vi "Test Database API.vi"() -> ()   [LabVIEW 2016]
doc: "Database API Tester."
uses:
  Class/DB/Credential.ctl
  Class/DB/Update Credential.ctl
  <vilib>/Utility/error.llb/DialogType.ctl
  Database.lvlib
panel:
  in  "REQ Retry DB":bool
  in  "REQ Close DB Ref":bool
  in  "User Level":enum16{"Administrator", "Engineer", "Operator"}(ring)
  out "Username":string[](array[string])
  in  "REQ Get Username":bool
  out "Test Data Out":string[][](array[string])
  in  "To":timestamp
  in  "From":timestamp
  in  "REQ Load Test Data":bool
  in  "Test Data":string[](array[string])
  in  "REQ Save Test Data":bool
  in  "REQ Save DB Record Data":bool
  in  "REQ Delete Table Data":bool
  in  "List Table":string(combo)
  in  "REQ List Table":bool
  in  "New Credential":T1
  in  "REQ Update User Details":bool
  in  "REQ Delete User":bool
  out "Match?":bool
  in  "REQ Check Credential":bool
  in  "Credential":T2
  in  "REQ Add User":bool
  in  "Show Diagram on Init":bool
  in  "Show Block Diagram":bool
  in  "Stop Module":bool
  in  "Start Module":bool
  in  "Hide Module Panel":bool
  in  "Show Module Panel":bool
  out "Status":string
  out "Module Running?":bool
  # "This VI tests the API for the Module."
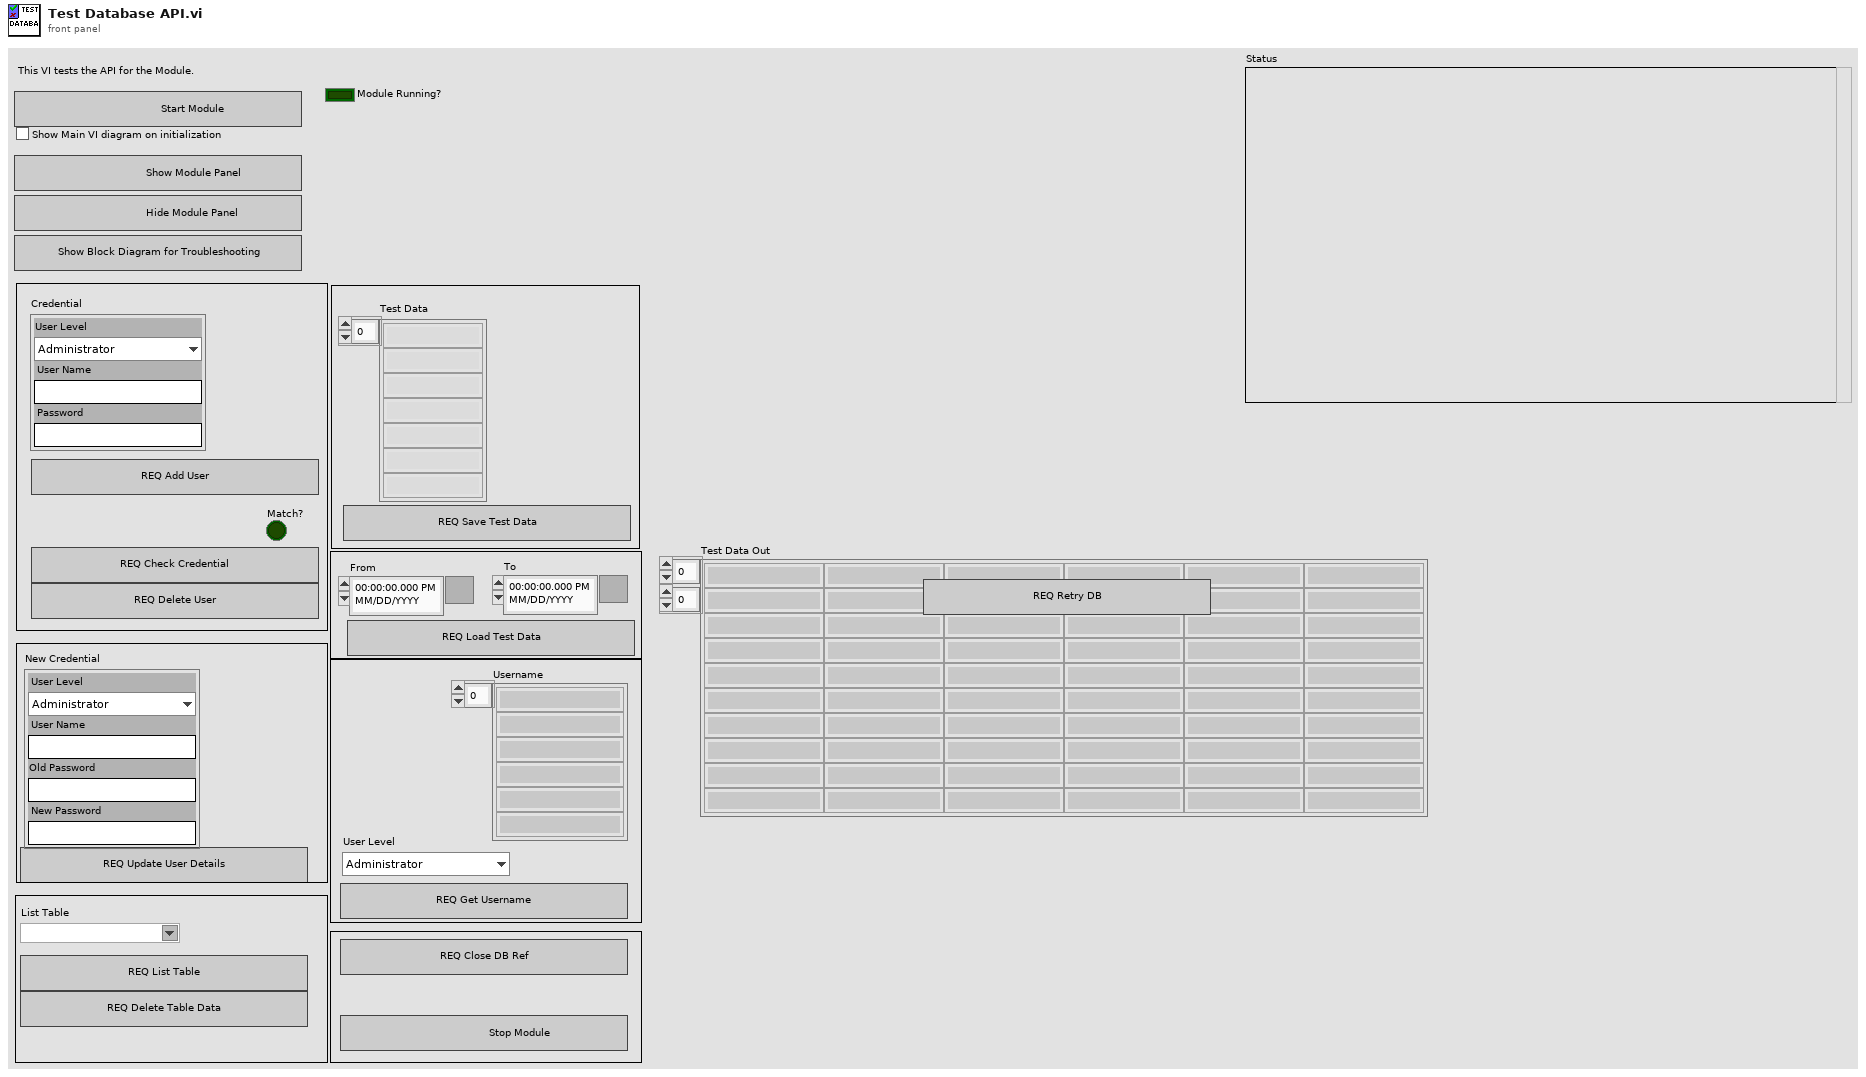
[diagram p1: front panel]
types:
  T1 = typedef "Database.lvlib/Update Credential.ctl" = cluster{"User Level":enum16{"Administrator", "Engineer", "Operator"}, "User Name":string, "Old Password":string, "New Password":string}
  T2 = typedef "Database.lvlib/Credential.ctl" = cluster{"User Level":enum16{"Administrator", "Engineer", "Operator"}, "User Name":string, "Password":string}
  T3 = typedef "Database.lvlib/Broadcast Events--cluster.ctl" = cluster{"Module Did Init":refnum<user-event>, "Status Updated":refnum<user-event>, "Error Reported":refnum<user-event>, "Module Did Stop":refnum<user-event>, "Update Module Execution Status":refnum<user-event>}
  T4 = typedef "DialogType.ctl" = u16
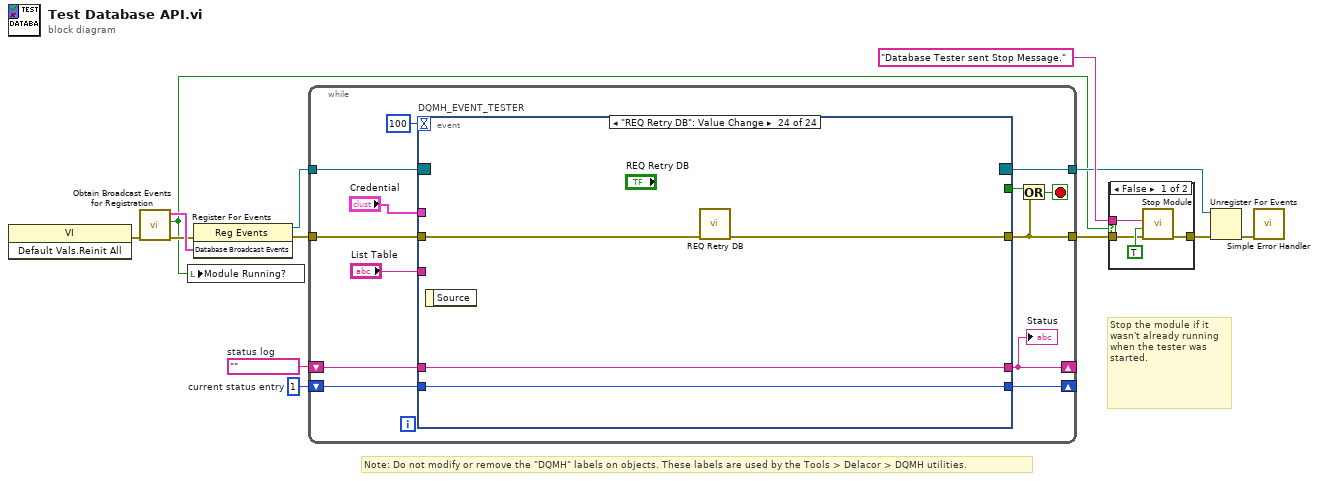
[diagram p0: block diagram]
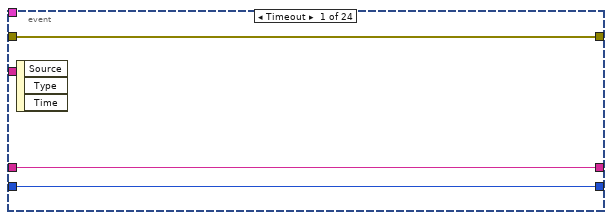
[diagram p3: hidden frame]
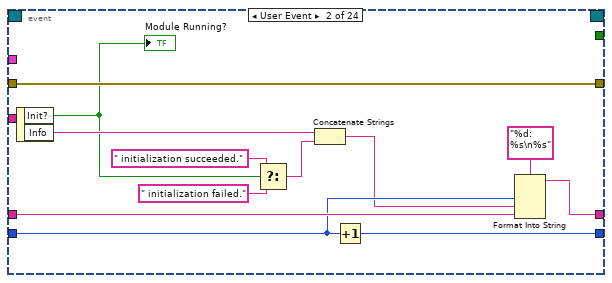
[diagram p4: hidden frame]
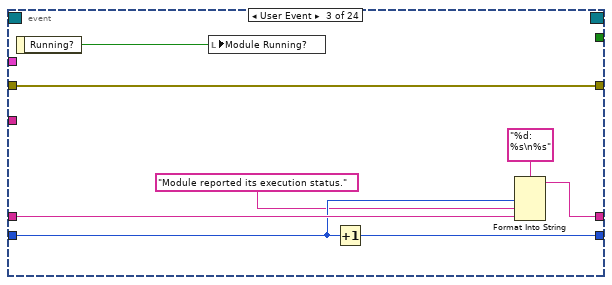
[diagram p5: hidden frame]
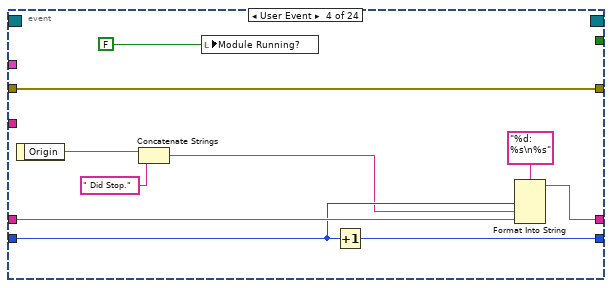
[diagram p6: hidden frame]
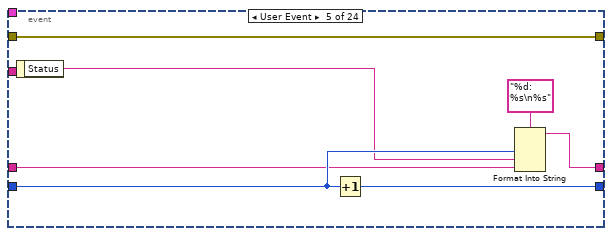
[diagram p7: hidden frame]
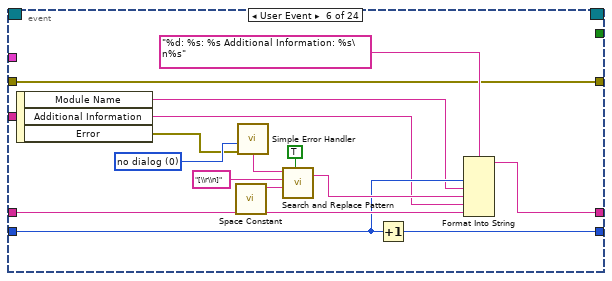
[diagram p8: hidden frame]
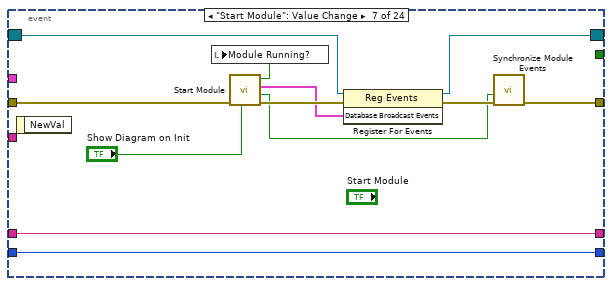
[diagram p9: hidden frame]
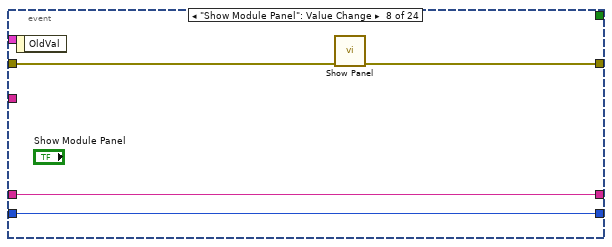
[diagram p10: hidden frame]
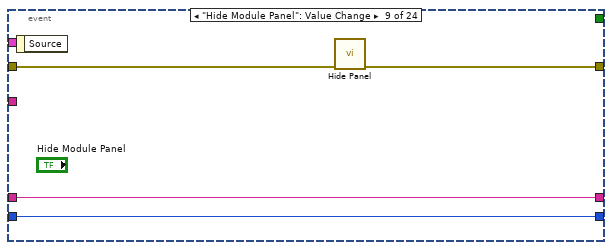
[diagram p11: hidden frame]
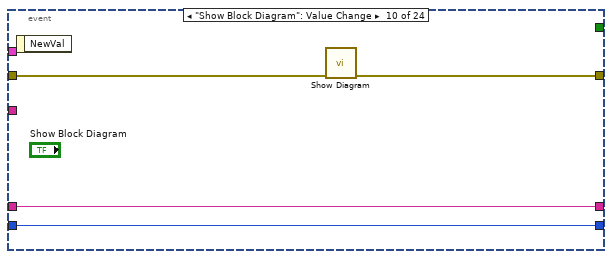
[diagram p12: hidden frame]
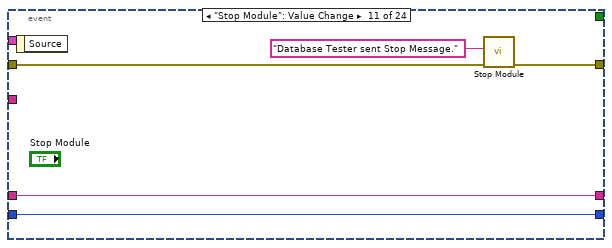
[diagram p13: hidden frame]
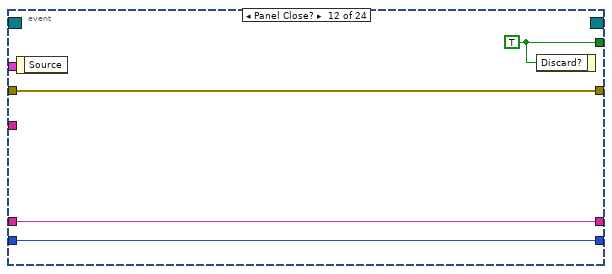
[diagram p14: hidden frame]
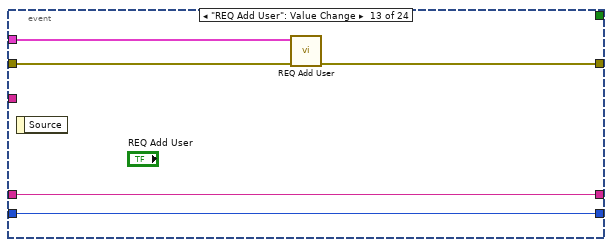
[diagram p15: hidden frame]
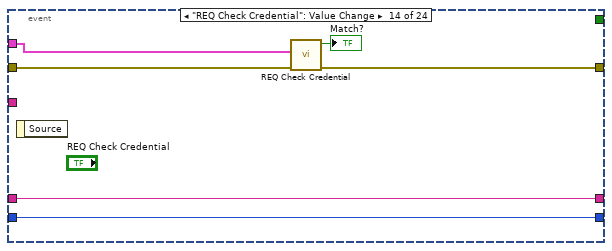
[diagram p16: hidden frame]
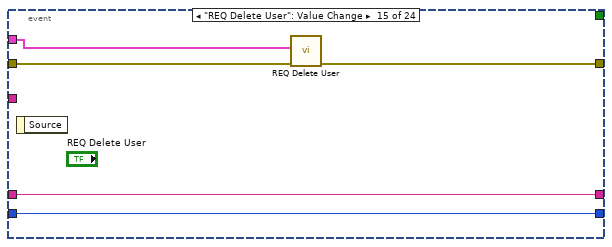
[diagram p17: hidden frame]
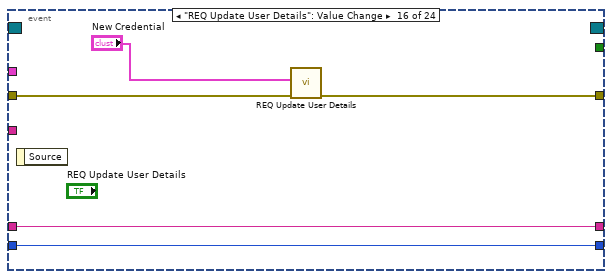
[diagram p18: hidden frame]
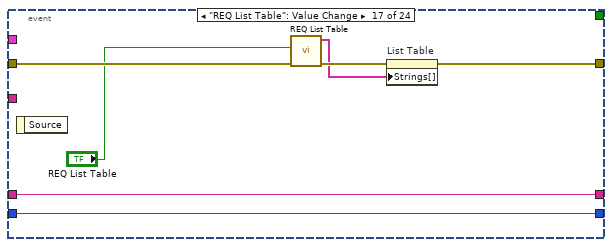
[diagram p19: hidden frame]
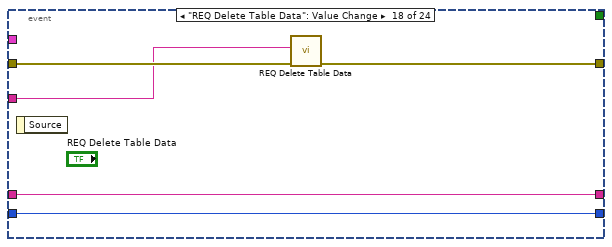
[diagram p20: hidden frame]
diagram:
  w10 = 1  # current status entry
  w11 = ""  # status log
  # "Stop the module if it wasn't already running when the tester was started."
  # "Note: Do not modify or remove the \"DQMH\" labels on objects. These labels are used by the Tools > Delacor > DQMH utilities."
  n1 = invoke class="VI" method="Default Vals.Reinit All"() -> (error out=w5:errorcluster)  [unwired: 3 in, 2 out]
  n2 = call "Obtain Broadcast Events for Registration.vi"("error in"=w5) -> ("error out"=w4:errorcluster, "Already running?"=w3:bool, "Database Broadcast Events"=w8:T3)  [unwired: 8 in]
  n3 = local write "Module Running?"(w3) -> ()
  n4 = register-events(error in=w4, w8) -> (reference out=w7:refnum<event-registration>, error out=w9:errorcluster)  [unwired: 1 in]
  n5 = while {
    tunnel: w7 -> [w26]
    tunnel: [w17] -> w2
    shift-right: [w21] -> _
    shift-left: w11 -> [w23]
    shift-right: [w22] -> _
    shift-left: w10 -> [w24]
    tunnel: w9 -> [w19]
    tunnel: [w18] -> w6
    stop <- w20 stop-if-true
    n6 = event "DQMH_EVENT_TESTER" shown="[23] \"REQ Retry DB\": Value Change" {
      selector: w26 -> [_ _ _ _ _ _ w87 _ _ _ _ _ _ _ _ _ _ _ _ _ _ _ _ _]
      dyn-events: [_ _ _ _ _ _ w86 _ _ _ _ _ _ _ _ _ _ _ _ _ _ _ _ _] -> w18
      timeout: 100 -> [_ _ _ _ _ _ _ _ _ _ _ _ _ _ _ _ _ _ _ _ _ _ _ _]
      tunnel: [_ _ _ _ _ _ _ _ _ _ _ w114 _ _ _ _ _ _ _ _ _ _ _ _] -> w25
      tunnel: [w29 w41 w43 w50 w60 w70 w85 w97 w101 w102 w108 w111 w116 w122 w127 w132 w137 w144 w148 w153 w160 w167 w171 w175] -> w17
      tunnel: w24 -> [w27 w38 w47 w57 w63 w73 w90 w95 w99 w103 w109 w112 w117 w123 w128 w133 w140 w145 w149 w154 w161 w168 w172 w176]
      tunnel: w23 -> [w28 w39 w48 w58 w62 w74 w91 w96 w100 w104 w110 w113 w118 w124 w129 w134 w141 w146 w150 w155 w162 w169 w173 w177]
      tunnel: [w28 w36 w45 w55 w64 w72 w91 w96 w100 w104 w110 w113 w118 w124 w129 w134 w141 w146 w150 w155 w162 w169 w173 w177] -> w21
      tunnel: [w27 w37 w46 w56 w66 w71 w90 w95 w99 w103 w109 w112 w117 w123 w128 w133 w140 w145 w149 w154 w161 w168 w172 w176] -> w22
      tunnel: w19 -> [w29 w41 w43 w50 w60 w70 w84 w94 w98 w105 w106 w111 w119 w125 w130 w135 w142 w147 w151 w156 w163 w170 w174 w178]
      tunnel: "Credential" -> [_ _ _ _ _ _ _ _ _ _ _ _ w115 w121 w126 _ _ _ _ _ _ w166 _ _]
      tunnel: "List Table" -> [_ _ _ _ _ _ _ _ _ _ _ _ _ _ _ _ _ w143 _ _ _ _ _ _]
      event Timeout {
        n7 = event-data() -> ()  [unwired: 1 in, 3 out]
      }
      event User Event {
        n8 = event-data() -> ("Init?"=w33:bool, "Info"=w35:string)  [unwired: 1 in]
        "Module Running?" <- w33
        n9 = Select(t=" initialization succeeded.", s=w33, f=" initialization failed.") -> (s? t:f=w30:string)
        n10 = Concatenate Strings(w35, w30) -> (w34:string)
        n11 = Increment(x=w38) -> (x+1=w37:i32)
        n12 = Format Into String(format string="%d: %s\n%s", w38, w34, w39) -> (resulting string=w36:string)  [unwired: 2 in, 1 out]
      }
      event User Event {
        n13 = event-data() -> ("Running?"=w42:bool)  [unwired: 1 in]
        n14 = local write "Module Running?"(w42) -> ()
        n15 = Increment(x=w47) -> (x+1=w46:i32)
        n16 = Format Into String(format string="%d: %s\n%s", w47, "Module reported its execution status.", w48) -> (resulting string=w45:string)  [unwired: 2 in, 1 out]
      }
      event User Event {
        n17 = event-data() -> ("Origin"=w54:string)  [unwired: 1 in]
        n18 = Concatenate Strings(w54, " Did Stop.") -> (w53:string)
        n19 = local write "Module Running?"(FALSE ("Module Did Init?")) -> ()
        n20 = Increment(x=w57) -> (x+1=w56:i32)
        n21 = Format Into String(format string="%d: %s\n%s", w57, w53, w58) -> (resulting string=w55:string)  [unwired: 2 in, 1 out]
      }
      event User Event {
        n22 = event-data() -> ("Status"=w61:string)  [unwired: 1 in]
        n23 = Increment(x=w63) -> (x+1=w66:i32)
        n24 = Format Into String(format string="%d: %s\n%s", w63, w61, w62) -> (resulting string=w64:string)  [unwired: 2 in, 1 out]
      }
      event User Event {
        w75 = T4 0 items=["no dialog", "OK message", "continue or stop message", "OK message + warnings", "continue/stop + warnings"] ("type of dialog (OK msg:1)")
        n25 = event-data() -> ("Module Name"=w69:string, "Additional Information"=w68:string, "Error"=w67:errorcluster)  [unwired: 1 in]
        n26 = call <vilib>:"Space Constant.vi"() -> ("String"=w79:string)
        n27 = call <vilib>:"Simple Error Handler.vi"("type of dialog (OK msg:1)"=w75, "error in (no error)"=w67) -> ("message"=w76:string)  [unwired: 3 in, 4 out]
        n28 = call <vilib>:"Search and Replace Pattern.vi"("string"=w76, "regular expression (\"\")"="[\\r\\n]" ("regular expression (\"\")"), "replace string (\"\")"=w79, "replace all? (F)"=TRUE ("replace all CR/LF with spaces")) -> ("result string"=w77:string)  [unwired: 1 in, 1 out]
        n29 = Increment(x=w73) -> (x+1=w71:i32)
        n30 = Format Into String(format string="%d: %s: %s Additional Information: %s\n%s", w73, w69, w77, w68, w74) -> (resulting string=w72:string)  [unwired: 2 in, 1 out]
      }
      event "Start Module": Value Change {
        n31 = event-data() -> ()  [unwired: 1 in, 1 out]
        n32 = call "Start Module.vi"("Show Main VI Diagram on Init (F)"="Show Diagram on Init", "error in"=w84) -> ("error out"=w92:errorcluster, "Wait for Event Sync?"=w89:bool, "Database Broadcast Events"=w88:T3, "Module Was Already Running?"=w83:bool)  [unwired: 6 in]
        n33 = local write "Module Running?"(w83) -> ()
        n34 = register-events(reference=w87, error in=w92, w88) -> (reference out=w86:refnum<event-registration>, error out=w93:errorcluster)
        n35 = call "Synchronize Module Events.vi"("error in"=w93, "Wait for Event Sync?"=w89) -> ("error out"=w85:errorcluster)  [unwired: 9 in]
      }
      event "Show Module Panel": Value Change {
        n36 = event-data() -> ()  [unwired: 1 in, 1 out]
        n37 = call "Show Panel.vi"("error in (no error)"=w94) -> ("error out"=w97:errorcluster)  [unwired: 10 in]
      }
      event "Hide Module Panel": Value Change {
        n38 = event-data() -> ()  [unwired: 1 in, 1 out]
        n39 = call "Hide Panel.vi"("error in (no error)"=w98) -> ("error out"=w101:errorcluster)  [unwired: 10 in]
      }
      event "Show Block Diagram": Value Change {
        n40 = event-data() -> ()  [unwired: 1 in, 1 out]
        n41 = call "Show Diagram.vi"("error in (no error)"=w105) -> ("error out"=w102:errorcluster)  [unwired: 10 in]
      }
      event "Stop Module": Value Change {
        n42 = event-data() -> ()  [unwired: 1 in, 1 out]
        n43 = call "Stop Module.vi"("error in"=w106, "Origin"="Database Tester sent Stop Message.") -> ("error out"=w108:errorcluster)  [unwired: 9 in]
      }
      event Panel Close? {
        w114 = TRUE ("Discard?")
        n44 = event-data() -> ()  [unwired: 1 in, 1 out]
        n45 = event-data("Discard?"=w114) -> ()  [unwired: 1 in, 1 out]
      }
      event "REQ Add User": Value Change {
        n46 = event-data() -> ()  [unwired: 1 in, 1 out]
        n47 = call "REQ Add User.vi"("error in"=w119, "Credential"=w115) -> ("error out"=w116:errorcluster)  [unwired: 9 in]
      }
      event "REQ Check Credential": Value Change {
        n48 = event-data() -> ()  [unwired: 1 in, 1 out]
        n49 = call "REQ Check Credential.vi"("error in"=w125, "Credential"=w121) -> ("error out"=w122:errorcluster, "Match?"=→"Match?":bool)  [unwired: 7 in, 1 out]
      }
      event "REQ Delete User": Value Change {
        n50 = event-data() -> ()  [unwired: 1 in, 1 out]
        n51 = call "REQ Delete User.vi"("error in"=w130, "Credential"=w126) -> ("error out"=w127:errorcluster)  [unwired: 9 in]
      }
      event "REQ Update User Details": Value Change {
        n52 = event-data() -> ()  [unwired: 1 in, 1 out]
        n53 = call "REQ Update User Details.vi"("error in"=w135, "Update Credential"="New Credential") -> ("error out"=w132:errorcluster)  [unwired: 9 in]
      }
      event "REQ List Table": Value Change {
        n54 = event-data() -> ()  [unwired: 1 in, 1 out]
        n55 = call "REQ List Table.vi"("error in"=w142, "Table?"="REQ List Table") -> ("error out"=w138:errorcluster, "List Table"=w136:string[])  [unwired: 7 in, 1 out]
        n56 = property on="List Table" class="CmbBox"(error in=w138, "Strings[]"=w136) -> (error out=w137:errorcluster)  [unwired: 1 in, 1 out]
      }
      event "REQ Delete Table Data": Value Change {
        n57 = event-data() -> ()  [unwired: 1 in, 1 out]
        n58 = call "REQ Delete Table Data.vi"("error in"=w147, "Table name"=w143) -> ("error out"=w144:errorcluster)  [unwired: 9 in]
      }
      event "REQ Save DB Record Data": Value Change {
        n59 = event-data() -> ()  [unwired: 1 in, 1 out]
        n60 = call "REQ Save DB Record Data.vi"("error in"=w151) -> ("error out"=w148:errorcluster)  [unwired: 10 in]
      }
      event "REQ Save Test Data": Value Change {
        n61 = event-data() -> ()  [unwired: 1 in, 1 out]
        n62 = call "REQ Save Test Data.vi"("error in"=w156, "Test Data"="Test Data") -> ("error out"=w153:errorcluster)  [unwired: 9 in]
      }
      event "REQ Load Test Data": Value Change {
        n63 = event-data() -> ()  [unwired: 1 in, 1 out]
        n64 = call "REQ Load Test Data.vi"("error in"=w163, "To"="To", "From"="From") -> ("error out"=w160:errorcluster, "Test Data"=→"Test Data Out":string[][])  [unwired: 6 in, 1 out]
      }
      event "REQ Get Username": Value Change {
        n65 = event-data() -> ()  [unwired: 1 in, 1 out]
        n66 = Unbundle By Name(w166) -> ()  [unwired: 1 out]
        n67 = call "REQ Get Username.vi"("error in"=w170, "User Level"="User Level") -> ("error out"=w167:errorcluster, "Username"=→"Username":string[])  [unwired: 7 in, 1 out]
      }
      event "REQ Close DB Ref": Value Change {
        n68 = event-data() -> ()  [unwired: 1 in, 1 out]
        n69 = call "REQ Close DB Ref.vi"("error in"=w174) -> ("error out"=w171:errorcluster)  [unwired: 10 in]
      }
      event "REQ Retry DB": Value Change {
        n70 = event-data() -> ()  [unwired: 1 in, 1 out]
        n71 = call "REQ Retry DB.vi"("error in"=w178) -> ("error out"=w175:errorcluster)  [unwired: 10 in]
      }
    }
    "Status" <- w21
    n72 = Or(x=w25, y=w17) -> (x .or. y?=w20:bool)
  }
  n73 = case shown="False" w3 {
    tunnel: [w182 w183] -> w13
    tunnel: "Database Tester sent Stop Message." ("Origin") -> [w181 _]
    tunnel: w2 -> [w179 w183]
    frame False {
      n74 = call "Stop Module.vi"("error in"=w179, "Wait for Module to Stop? (F)"=TRUE ("Wait for Module to stop?"), "Origin"=w181) -> ("error out"=w182:errorcluster)  [unwired: 8 in]
    }
    frame True {
    }
  }
  n75 = Unregister For Events(event registration refnum=w6, error in=w13) -> (error out=w1:errorcluster)
  n76 = call <vilib>:"Simple Error Handler.vi"("error in (no error)"=w1) -> ()  [unwired: 4 in, 5 out]
